vi "Test Equipment - Servo and Force.vi"(7 "fs notifier":refnum<notifier>, 8 "error in (no error)":errorcluster, 9 "gui notifier":refnum<notifier>, 10 "error queue":refnum<queue>, 11 "servo queue":refnum<queue>) -> (0 "error out":errorcluster)   [LabVIEW 2020]
uses:
  Hardware/Actuators/Servos/Servo.lvclass
  C:/Users/jharw/Documents/1 Folder to Rule them All/UMD/Inflation-Apparatus/src/Hardware/General Hardware.lvclass
  Main GUI Loop/Handler.ctl
  Hardware/Sensors/Force Sensors/Force Sensor.lvclass
  Hardware/Actuators/Servos/Servo.lvclass/Servo.ctl
  Hardware/General Hardware.lvclass/General Hardware.ctl
  Hardware/Sensors/Force Sensors/Force Sensor.lvclass/Force Sensor.ctl
  Hardware/General Hardware.lvclass
panel:
  out "current force":dbl(graph)
  in  "servo slider":dbl(slide)=1400.0 caption="SERVO POSITION" min=800.0 max=2000.0 step=5.0 scale=800.0..2000.0
  # "CURRENT FORCE"
  # "SERVO PULSE-WIDTH POSITION (micro-sec)"
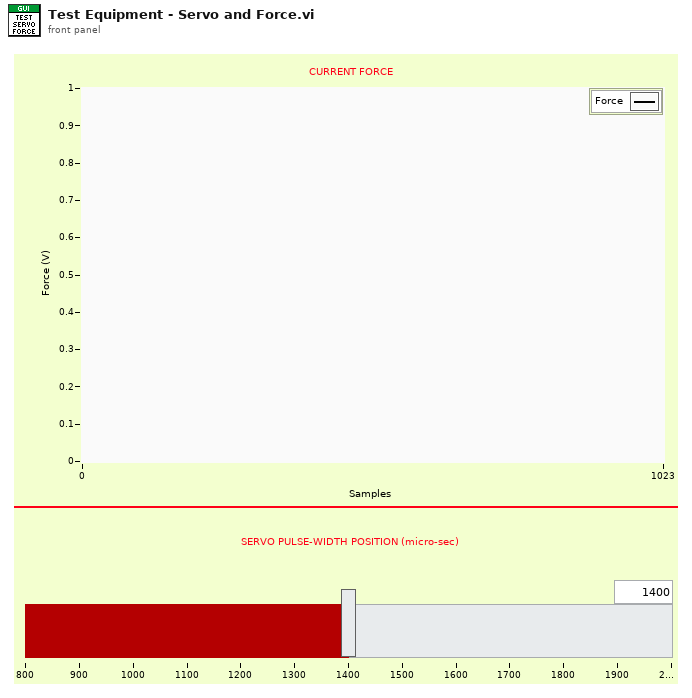
[diagram p1: front panel]
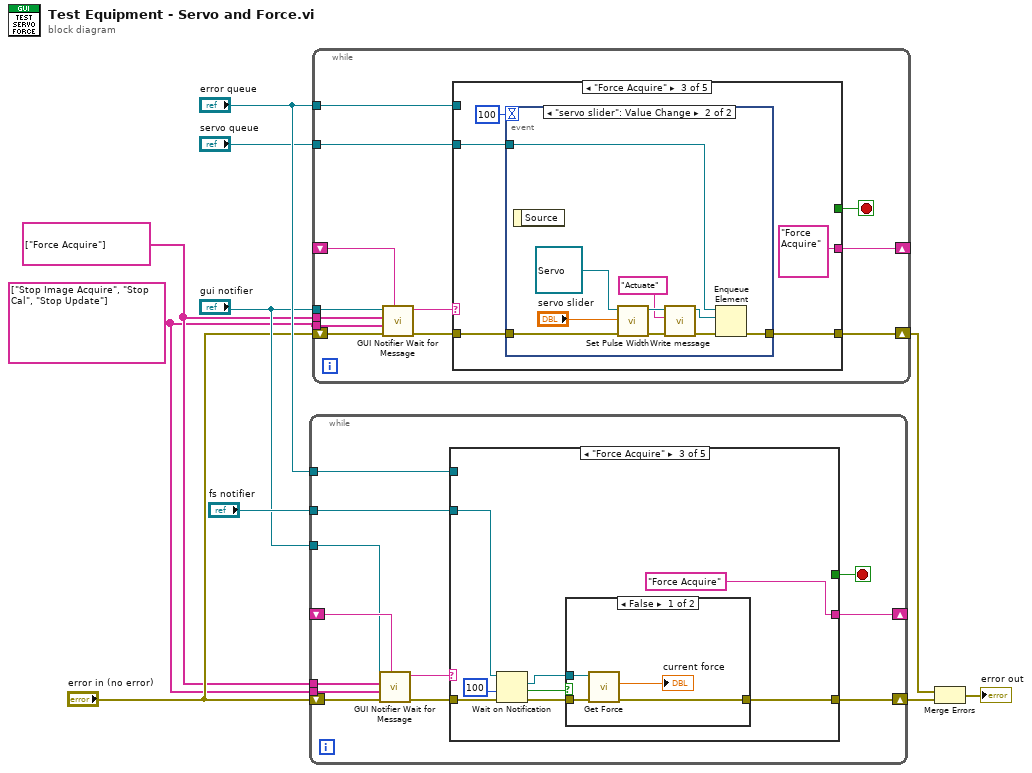
[diagram p0: block diagram]
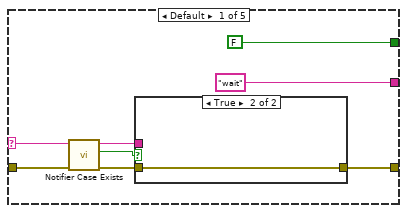
[diagram p2: hidden frame]
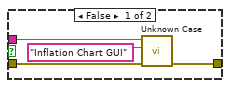
[diagram p3: hidden frame]
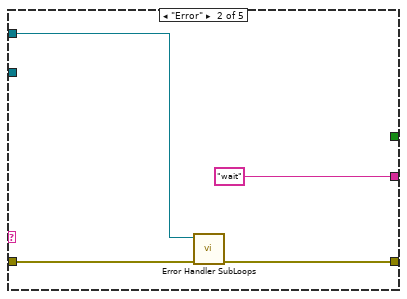
[diagram p4: hidden frame]
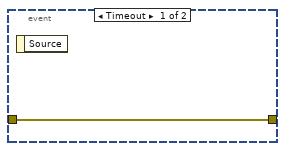
[diagram p5: hidden frame]
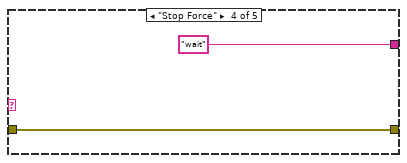
[diagram p6: hidden frame]
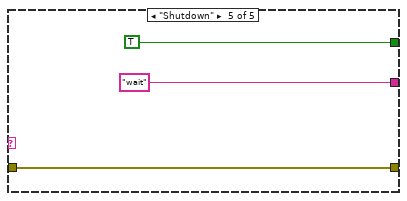
[diagram p7: hidden frame]
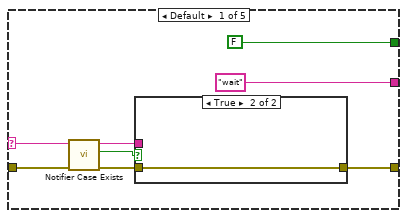
[diagram p8: hidden frame]
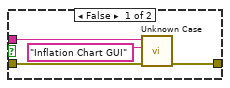
[diagram p9: hidden frame]
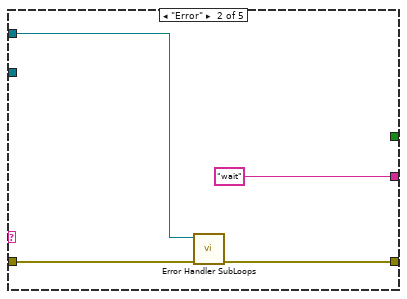
[diagram p10: hidden frame]
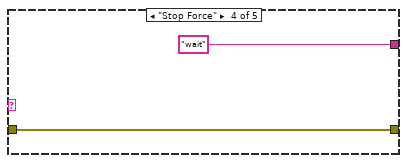
[diagram p12: hidden frame]
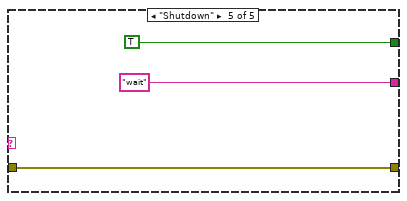
[diagram p13: hidden frame]
diagram:
  w1 = string[] ["Stop Image Acquire", "Stop Cal", "Stop Update"] ("notification")
  w2 = string[] ["Force Acquire"] ("t")
  n1 = while {
    tunnel: w1 -> [w20]
    tunnel: w2 -> [w19]
    shift-right: [w18] -> _
    shift-left: _ -> [w17]
    shift-right: [w15] -> w9
    shift-left: "error in (no error)" -> [w16]
    tunnel: "fs notifier" -> [w13]
    tunnel: "error queue" -> [w12]
    tunnel: "gui notifier" -> [w11]
    stop <- w14 stop-if-true
    n2 = call "GUI Notifier Wait for Message.vi"("last state"=w17, "error in (no error)"=w16, "cases to ignore"=w20, "acquisition states"=w19, "gui notifier"=w11) -> ("error out"=w21:errorcluster, "gui msg"=w22:string)  [unwired: 5 in]
    n3 = case shown="\"Force Acquire\"" w22 {
      selector: w22 -> [w28 _ _ _ _]
      tunnel: [FALSE _ _ _ TRUE] -> w14
      tunnel: w21 -> [w27 w39 w47 w53 w56]
      tunnel: [w29 w38 w43 w53 w56] -> w15
      tunnel: w12 -> [_ w37 _ _ _]
      tunnel: w13 -> [_ _ w45 _ _]
      tunnel: ["wait" "wait" "Force Acquire" "wait" "wait"] -> w18
      frame Default {
        n4 = call "Notifier Case Exists.vi"("error in (no error)"=w27, "case in"=w28) -> ("error out"=w26:errorcluster, "defined case?"=w24:bool, "case out"=w25:string)  [unwired: 7 in]
        n5 = case shown="True" w24 {
          tunnel: [w34 w35] -> w29
          tunnel: w26 -> [w32 w35]
          tunnel: w25 -> [w31 _]
          frame False {
            n6 = call "Unknown Case.vi"("error in (no error)"=w32, "source"="Inflation Chart GUI", "case"=w31) -> ("error out"=w34:errorcluster)  [unwired: 8 in]
          }
          frame True {
          }
        }
      }
      frame "Error" {
        n7 = call "Error Handler SubLoops.vi"("error in"=w39, "main gui queue"=w37) -> ("error out"=w38:errorcluster)  [unwired: 9 in]
      }
      frame "Force Acquire" {
        n8 = Wait on Notification(notifier=w45, timeout in ms (-1)=100, error in (no error)=w47) -> (notification=w42:refnum<class "Force Sensor.lvclass">, timed out?=w41:bool, error out=w44:errorcluster)  [unwired: 1 in, 1 out]
        n9 = case shown="False" w41 {
          tunnel: w44 -> [w51 w52]
          tunnel: [w50 w52] -> w43
          tunnel: w42 -> [w49 _]
          frame False {
            n10 = call "Get Force.vi"("error in (no error)"=w51, "Force Sensor in"=w49) -> ("error out"=w50:errorcluster, "force (V)"=→"current force":dbl)  [unwired: 7 in, 1 out]
          }
          frame True {
            # "Only update if not timed out"
          }
        }
      }
      frame "Stop Force" {
      }
      frame "Shutdown" {
      }
    }
  }
  n11 = while {
    shift-right: [w67] -> _
    shift-left: _ -> [w66]
    shift-right: [w64] -> w7
    shift-left: "error in (no error)" -> [w65]
    tunnel: "servo queue" -> [w62]
    tunnel: "error queue" -> [w61]
    tunnel: "gui notifier" -> [w60]
    tunnel: w2 -> [w59]
    tunnel: w1 -> [w58]
    stop <- w63 stop-if-true
    n12 = call "GUI Notifier Wait for Message.vi"("last state"=w66, "error in (no error)"=w65, "cases to ignore"=w58, "acquisition states"=w59, "gui notifier"=w60) -> ("error out"=w68:errorcluster, "gui msg"=w69:string)  [unwired: 5 in]
    n13 = case shown="\"Force Acquire\"" w69 {
      selector: w69 -> [w75 _ _ _ _]
      tunnel: [FALSE _ _ _ TRUE] -> w63
      tunnel: w68 -> [w74 w86 w88 w103 w106]
      tunnel: [w76 w85 w89 w103 w106] -> w64
      tunnel: w61 -> [_ w84 _ _ _]
      tunnel: w62 -> [_ _ w87 _ _]
      tunnel: ["wait" "wait" "Force Acquire" "wait" "wait"] -> w67
      frame Default {
        n14 = call "Notifier Case Exists.vi"("error in (no error)"=w74, "case in"=w75) -> ("error out"=w73:errorcluster, "defined case?"=w71:bool, "case out"=w72:string)  [unwired: 7 in]
        n15 = case shown="True" w71 {
          tunnel: [w81 w82] -> w76
          tunnel: w73 -> [w79 w82]
          tunnel: w72 -> [w78 _]
          frame False {
            n16 = call "Unknown Case.vi"("error in (no error)"=w79, "source"="Inflation Chart GUI", "case"=w78) -> ("error out"=w81:errorcluster)  [unwired: 8 in]
          }
          frame True {
          }
        }
      }
      frame "Error" {
        n17 = call "Error Handler SubLoops.vi"("error in"=w86, "main gui queue"=w84) -> ("error out"=w85:errorcluster)  [unwired: 9 in]
      }
      frame "Force Acquire" {
        n18 = event shown="[1] \"servo slider\": Value Change" {
          selector: _ -> [_ _]
          dyn-events: _ -> [_ _]
          timeout: 100 ("timeout in ms (-1)") -> [_ _]
          tunnel: [w92 w102] -> w89
          tunnel: w88 -> [w92 w100]
          tunnel: w87 -> [_ w101]
          event Timeout {
            n19 = event-data() -> ()  [unwired: 1 in, 1 out]
          }
          event "servo slider": Value Change {
            n20 = event-data() -> ()  [unwired: 1 in, 1 out]
            n21 = call "Set Pulse Width.vi"("error in (no error)"=w100, "pulse width (micro-sec)"="servo slider", "Servo in"=refnum<class "Servo.lvclass"> refnum) -> ("error out"=w97:errorcluster, "Servo out"=w95:refnum<class "Servo.lvclass">)  [unwired: 7 in]
            n22 = call "Write message.vi"("error in (no error)"=w97, "message"="Actuate", "General Hardware in"=w95) -> ("error out"=w96:errorcluster, "General Hardware out"=w94:refnum<class "Servo.lvclass">)  [unwired: 7 in]
            n23 = Enqueue Element(queue=w101, element=w94, error in (no error)=w96) -> (error out=w102:errorcluster)  [unwired: 1 in, 2 out]
          }
        }
      }
      frame "Stop Force" {
      }
      frame "Shutdown" {
      }
    }
  }
  n24 = Merge Errors(w7, w9) -> (→"error out":errorcluster)
